vi "writeToXML.vi"(8 "error in (no error)":errorcluster, 10 "ClassLAbel":string, 11 "TCSGuiderCommand.lvclass":refnum<class "TCSGuiderCommand.lvclass">) -> (0 "error out":errorcluster, 2 "XML out":string, 3 "TCSGuiderCommand.lvclass 2":refnum<class "TCSGuiderCommand.lvclass">)   [LabVIEW 2014, in "TCSDataDefinitions.lvlib" / "TCSGuiderCommand.lvlib" / "TCSGuiderCommand.lvclass"]
uses:
  TCSGuiderCommand.lvclass
  TCSCommand/TCSCommand/TCSCommand.lvclass
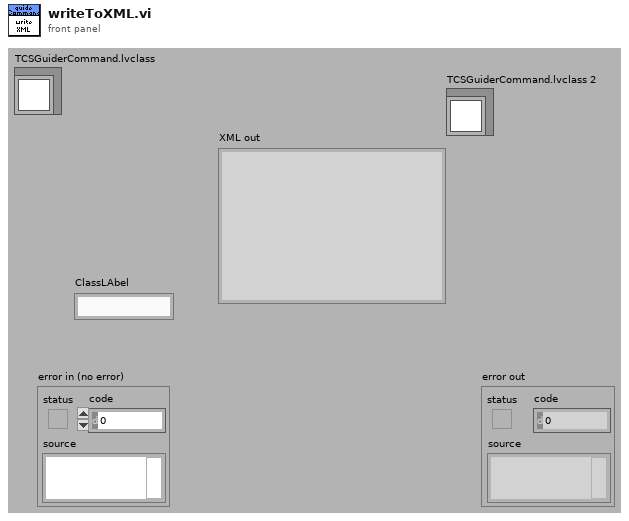
[diagram p1: front panel]
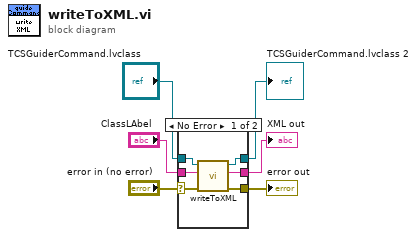
[diagram p0: block diagram]
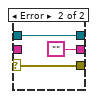
[diagram p2: hidden frame]
diagram:
  n1 = case shown="No Error" "error in (no error)" {
    selector: "error in (no error)" -> [w9 w15]
    tunnel: [w8 w15] -> w5
    tunnel: [w11 w14] -> w1
    tunnel: "TCSGuiderCommand.lvclass" -> [w12 w14]
    tunnel: "ClassLAbel" -> [w7 _]
    tunnel: [w10 ""] -> w3
    frame No Error {
      n2 = call-parent "writeToXML.vi"("error in (no error)"=w9, "Class Label"=w7, "TCSCommand in"=w12) -> ("error out"=w8:errorcluster, "XML out"=w10:string, "TCSCommand out"=w11:refnum<class "TCSGuiderCommand.lvclass">)  [unwired: 6 in]
    }
    frame Error {
    }
  }
  "error out" <- w5
  "XML out" <- w3
  "TCSGuiderCommand.lvclass 2" <- w1
